vi "Recompile directories.vi"(8 "error in":errorcluster, 10 "Directories":path[](array[path])) -> (0 "error out":errorcluster)   [LabVIEW 2010]
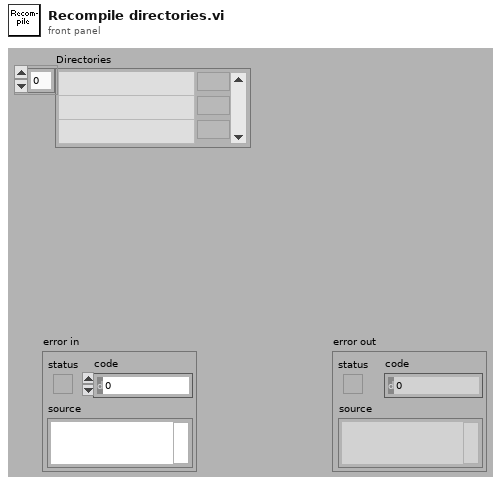
[diagram p1: front panel]
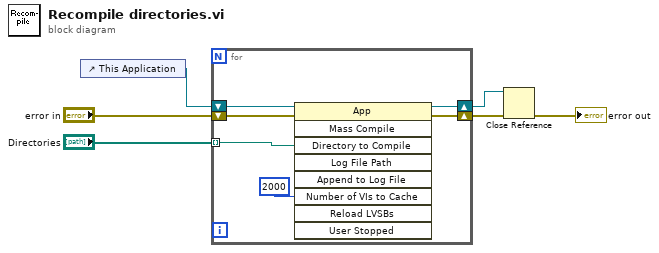
[diagram p0: block diagram]
diagram:
  n1 = control-ref of="This Application"() -> (w6:refnum<vi>)
  n2 = for {
    tunnel: "Directories" -> [w11] mode=indexing
    shift-right: [w10] -> w5
    shift-left: "error in" -> [w12]
    shift-right: [w8] -> w4
    shift-left: w6 -> [w9]
    n3 = invoke class="App" method="Mass Compile"(reference=w9, error in=w12, "Directory to Compile"=w11, "Number of VIs to Cache"=u32 2000) -> (reference out=w8:refnum<vi>, error out=w10:errorcluster)  [unwired: 5 in, 7 out]
  }
  n4 = Close Reference(reference=w4, error in (no error)=w5) -> (error out=→"error out":errorcluster)
